vi "Create Temp File.vi"(8 "Error In":errorcluster, 10 "Temp Settings File Contents (comments removed)":string, 11 "Temp Settings Filepath":path) -> (0 "Error Out":errorcluster)   [LabVIEW 2016, in "Error Manager.lvlib" / "Settings.lvclass"]
doc: "This VI creates a temporary file. This temp file contains the contents of the original settings file, minus any comments. A temp file is necessary because the built-in LabVIEW INI VIs take a filepath as an input (rather than a string).\n\nThe temp file will be deleted shortly after (milliseconds after)."
uses:
  Settings.lvclass
panel:
  # "Development\nControls or indicators that are useful for development or testing, but which are not outputs of the VI."
  # "Input\nInputs to the VI"
  # "Output\nOutputs of the VI"
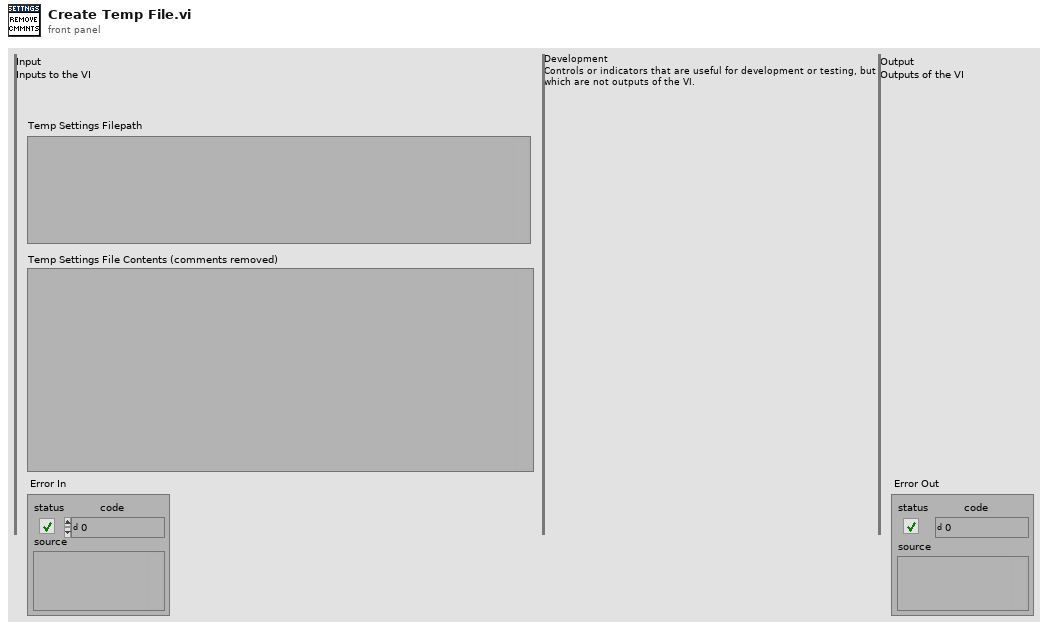
[diagram p1: front panel]
types:
  T1 = enum16{"open", "replace", "create", "open or create", "replace or create", "replace or create with confirmation"}
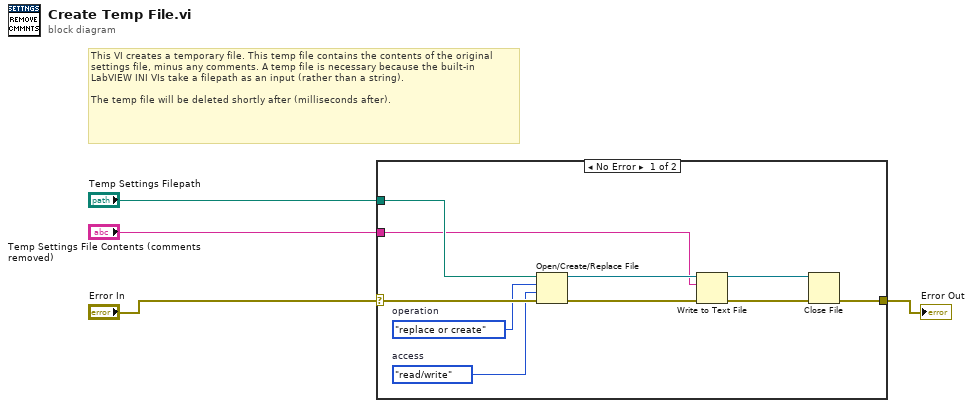
[diagram p0: block diagram]
diagram:
  # "This VI creates a temporary file. This temp file contains the contents of the original settings file, minus any comments. A temp file is necessary because the built-in LabVIEW INI VIs take a filepath as an input (rather than a string).\n\nThe temp file will be deleted shortly after (milliseconds after)."
  n1 = case shown="No Error" "Error In" {
    selector: "Error In" -> [w14 w15]
    tunnel: [w8 w15] -> w3
    tunnel: "Temp Settings Filepath" -> [w12 _]
    tunnel: "Temp Settings File Contents (comments removed)" -> [w5 _]
    frame No Error {
      w10 = enum16{"read/write", "read-only", "write-only"}."read/write"  # access
      w11 = T1."replace or create"  # operation
      n2 = Open/Create/Replace File(file path (use dialog)=w12, error in=w14, operation (0:open)=w11, access (0:read/write)=w10) -> (refnum out=w7:refnum<file>, error out=w13:errorcluster)  [unwired: 2 in, 1 out]
      n3 = Write to Text File(file (use dialog)=w7, text=w5, error in=w13) -> (refnum out=w6:refnum<file>, error out=w9:errorcluster)  [unwired: 1 in, 1 out]
      n4 = Close File(refnum=w6, error in=w9) -> (error out=w8:errorcluster)  [unwired: 1 out]
    }
    frame Error {
    }
  }
  "Error Out" <- w3
